vi "Write Compile Process Hook.vi"(8 "Error In":errorcluster, 10 "Compile Process":refnum<class "Process.lvclass">, 11 "Context In":refnum<class "Compiler.lvclass">) -> (0 "Error Out":errorcluster, 3 "Context Out":refnum<class "Compiler.lvclass">)   [LabVIEW 2018, in "Toolkit.lvlib" / "Compiler.lvclass"]
uses:
  Compiler.lvclass
  Hooks/Compile/Process/Process.lvclass
  Compiler.lvclass/Compiler.ctl
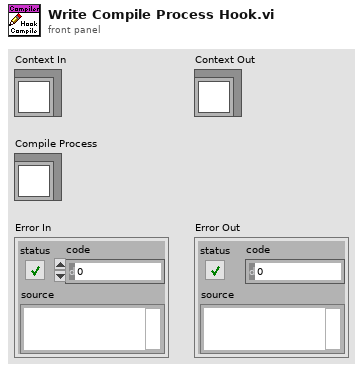
[diagram p1: front panel]
types:
  T1 = typedef "Toolkit.lvlib/Hooks.ctl" = cluster{"Compile":cluster{"Process":refnum<class "Process.lvclass">}, "Render":cluster{"Comment":refnum<class "Comment.lvclass">, "Delimiter":refnum<class "Delimiter.lvclass">, "Node":refnum<class "Node.lvclass">, "Partial":refnum<class "Partial.lvclass">, "Process":refnum<class "Process.lvclass">, "Section":refnum<class "Section.lvclass">, "Text":refnum<class "Text.lvclass">, "Variable":refnum<class "Variable.lvclass">}}
  T2 = cluster{"Process":refnum<class "Process.lvclass">}
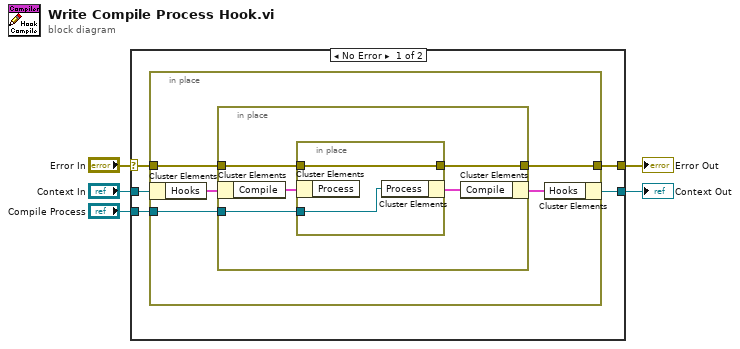
[diagram p0: block diagram]
diagram:
  n1 = case shown="No Error" "Error In" {
    selector: "Error In" -> [w7 w24]
    tunnel: "Context In" -> [w10 w23]
    tunnel: [w6 w24] -> w3
    tunnel: [w9 w23] -> w2
    tunnel: "Compile Process" -> [w8 _]
    frame No Error {
      n2 = in-place {
        in-place-border: w8 -> [w13]
        in-place-border: w7 -> [w12]
        in-place-border: [w11] -> w6
        n3 = in-place-cluster #1(w10) -> ("Hooks"=w15:T1)
        n4 = in-place {
          in-place-border: w13 -> [w18]
          in-place-border: w12 -> [w17]
          in-place-border: [w16] -> w11
          n5 = in-place-cluster #2(w15) -> ("Compile"=w20:T2)
          n6 = in-place {
            in-place-border: w18 -> [w22]
            in-place-border: w17 -> [w21]
            in-place-border: [w21] -> w16
            n7 = in-place-cluster #3(w20) -> ()  [unwired: 1 out]
            n8 = in-place-cluster #3("Process"=w22) -> (w19:T2)
          }
          n9 = in-place-cluster #2("Compile"=w19) -> (w14:T1)
        }
        n10 = in-place-cluster #1("Hooks"=w14) -> (w9:refnum<class "Compiler.lvclass">)
      }
    }
    frame Error {
    }
  }
  "Error Out" <- w3
  "Context Out" <- w2
